vi "Tracepoint_ServerError.vi"(8 "error in (no error)":errorcluster, 9 "String":string, 10 "Error":bool, 11 "Qbus":refnum<class "Qbus.lvclass">) -> (0 "error out":errorcluster)   [LabVIEW 2017, in "ModbusMaster.lvlib"]
uses:
  <vilib>/addons/Qbus/Qbus.lvclass
  <vilib>/addons/InsightCM/Devices/Shared/Common/ModbusMaster/ModbusMaster.lvlib
  <vilib>/addons/TraceLogger/TraceLogger.lvlib
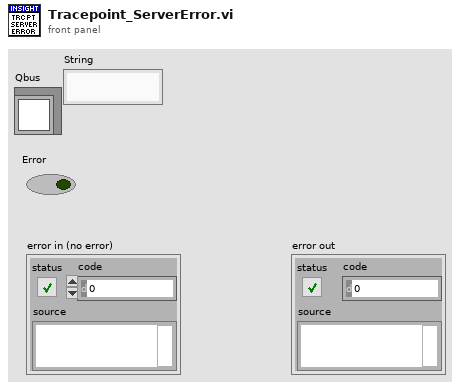
[diagram p1: front panel]
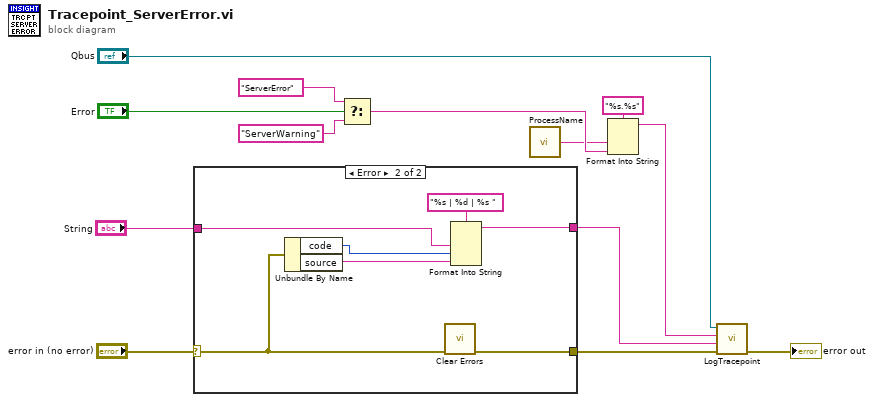
[diagram p0: block diagram]
diagram:
  n1 = case shown="Error" "error in (no error)" {
    selector: "error in (no error)" -> [w15 w19]
    tunnel: [w15 w22] -> w5
    tunnel: [w14 w20] -> w4
    tunnel: "String" -> [w14 w16]
    frame No Error {
    }
    frame Error {
      n2 = Unbundle By Name(w19) -> ("code"=w18:i32, "source"=w17:string)
      n3 = call <vilib>:"Clear Errors.vi"("error in (no error)"=w19) -> ("error out"=w22:errorcluster)  [unwired: 5 in, 1 out]
      n4 = Format Into String(format string="%s | %d | %s ", w16, w18, w17) -> (resulting string=w20:string)  [unwired: 2 in, 1 out]
    }
  }
  n5 = Select(t="ServerError" ("tracepoint"), s="Error", f="ServerWarning" ("tracepoint")) -> (s? t:f=w7:string)
  n6 = call <vilib>:"ProcessName.vi"() -> ("process name"=w1:string)  [unwired: 5 in]
  n7 = Format Into String(format string="%s.%s", w1, w7) -> (resulting string=w6:string)  [unwired: 2 in, 1 out]
  n8 = call <vilib>:"LogTracepoint.vi"("error in (no error)"=w5, "log string"=w4, "tracepoint"=w6, "qbus in"="Qbus") -> ("error out"=→"error out":errorcluster)  [unwired: 6 in, 1 out]
